vi "Agilent VNA Set Number of Points.vi"(6 "Channel":i8=1 min=1 max=99 step=1, 7 "Agilent VNA":T1, 8 "error in (no error)":errorcluster, 10 "Number Points":i32, 11 "VISA Resource Name":refnum<visa-resource-name>) -> (0 "error out":errorcluster, 3 "dup VISA Resource Name":refnum<visa-resource-name>)   [LabVIEW 2011]
doc: "This VI for the HP 8753B is used to read the number of stimulus points."
uses:
  TypeDefs/Agilent VNA Instrument Info.ctl
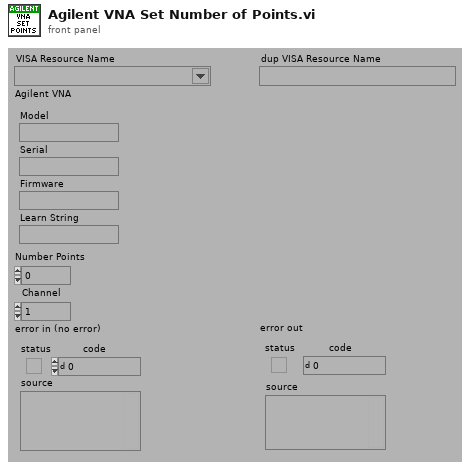
[diagram p1: front panel]
types:
  T1 = typedef "Agilent VNA Instrument Info.ctl" = cluster{"Model":string, "Serial":string, "Firmware":string, "Learn String":string}
  T2 = typedef "Agilent VNA Model.ctl" = enum16{"Not Supported", "8510X", "8719X", "8720X", "8722X", "8753X", "ENA", "PNA", "Field Fox"}
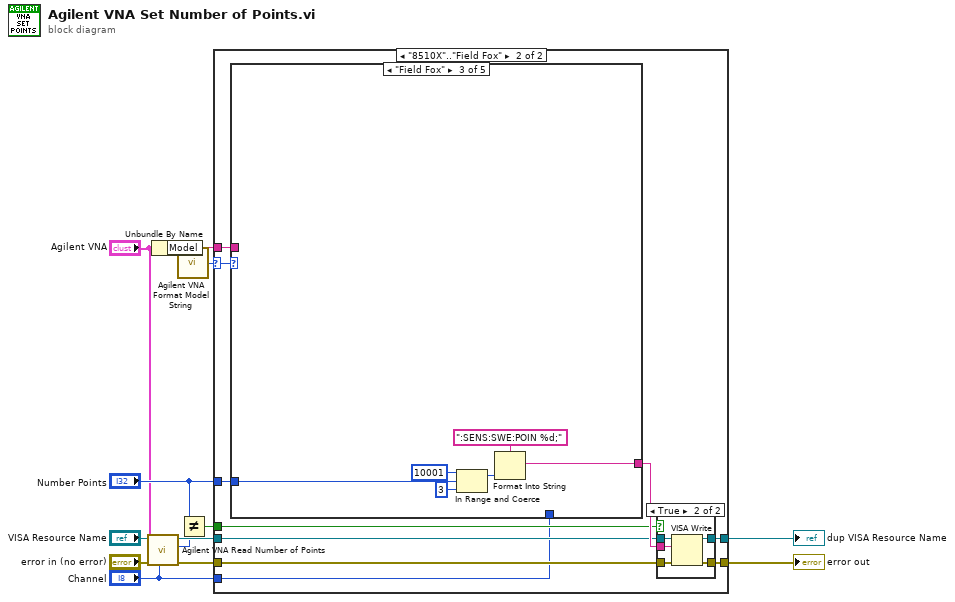
[diagram p0: block diagram]
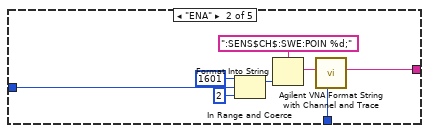
[diagram p4: hidden frame]
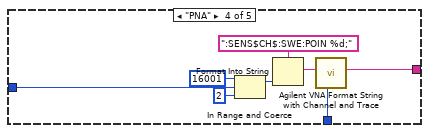
[diagram p5: hidden frame]
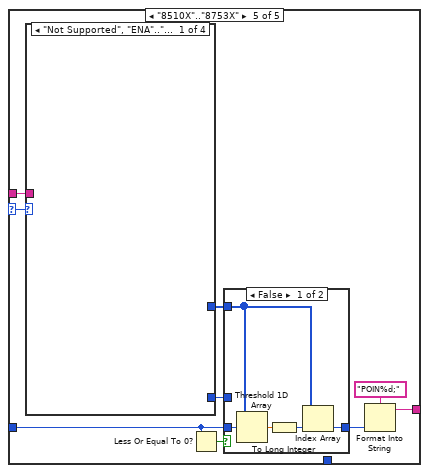
[diagram p6: hidden frame]
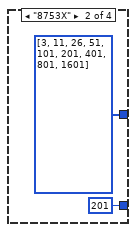
[diagram p8: hidden frame]
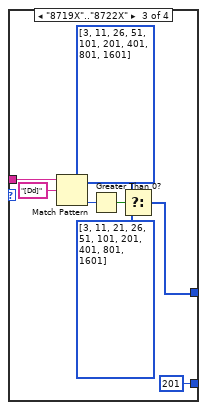
[diagram p9: hidden frame]
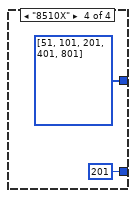
[diagram p10: hidden frame]
diagram:
  n1 = call "Agilent VNA Read Number of Points.vi"("Channel"="Channel", "Agilent VNA"="Agilent VNA", "error in (no error)"="error in (no error)", "VISA Resource Name"="VISA Resource Name") -> ("error out"=w6:errorcluster, "Number Points"=w5:i32, "dup VISA Resource Name"=w7:refnum<visa-resource-name>)  [unwired: 5 out]
  n2 = Unbundle By Name("Agilent VNA") -> ("Model"=w1:string)
  n3 = call "Agilent VNA Format Model String.vi"("Model"=w1) -> ("Model"=w2:T2)
  n4 = Not Equal?(x="Number Points", y=w5) -> (x != y?=w10:bool)
  n5 = case shown="\"8510X\"..\"Field Fox\"" w2 {
    selector: w2 -> [_ w17]
    tunnel: [w15 w25] -> w13
    tunnel: [w14 w24] -> w12
    tunnel: "Number Points" -> [_ w22]
    tunnel: w10 -> [_ w21]
    tunnel: w7 -> [w15 w20]
    tunnel: w6 -> [w14 w19]
    tunnel: "Channel" -> [_ w18]
    tunnel: w1 -> [_ w16]
    frame "Not Supported" {
    }
    frame "8510X".."Field Fox" {
      n6 = case shown="\"Field Fox\"" w17 {
        selector: w17 -> [_ _ _ _ w49]
        tunnel: [_ w27 w34 w41 w53] -> w23
        tunnel: w22 -> [_ w33 w39 w47 w50]
        tunnel: w18 -> [_ w26 _ w40 _]
        tunnel: w16 -> [_ _ _ _ w48]
        frame "Not Supported" {
        }
        frame "ENA" {
          n7 = In Range and Coerce(upper limit=1601, x=w33, lower limit=2) -> (coerced(x)=w29:i32)  [unwired: 1 out]
          n8 = Format Into String(format string=":SENS$CH$:SWE:POIN %d;", w29) -> (resulting string=w28:string)  [unwired: 2 in, 1 out]
          n9 = call "Agilent VNA Format String with Channel and Trace.vi"("Channel"=w26, "String"=w28) -> ("String Out"=w27:string)  [unwired: 1 in, 6 out]
        }
        frame "Field Fox" {
          n10 = In Range and Coerce(upper limit=10001, x=w39, lower limit=3) -> (coerced(x)=w35:i32)  [unwired: 1 out]
          n11 = Format Into String(format string=":SENS:SWE:POIN %d;", w35) -> (resulting string=w34:string)  [unwired: 2 in, 1 out]
        }
        frame "PNA" {
          n12 = In Range and Coerce(upper limit=16001, x=w47, lower limit=2) -> (coerced(x)=w43:i32)  [unwired: 1 out]
          n13 = Format Into String(format string=":SENS$CH$:SWE:POIN %d;", w43) -> (resulting string=w42:string)  [unwired: 2 in, 1 out]
          n14 = call "Agilent VNA Format String with Channel and Trace.vi"("Channel"=w40, "String"=w42) -> ("String Out"=w41:string)  [unwired: 1 in, 6 out]
        }
        frame "8510X".."8753X" {
          n15 = case shown="\"Not Supported\", \"ENA\"..\"Field Fox\"" w49 {
            tunnel: [_ i32[] [3, 11, 26, 51, 101, 201, 401, 801, 1601] w65 i32[] [51, 101, 201, 401, 801]] -> w55
            tunnel: [_ 201 201 201] -> w51
            tunnel: w48 -> [_ _ w70 _]
            frame "Not Supported", "ENA".."Field Fox" {
            }
            frame "8753X" {
            }
            frame "8719X".."8722X" {
              n16 = Match Pattern(string=w70, regular expression="[Dd]") -> (offset past match=w69:i32)  [unwired: 4 out]
              n17 = Greater Than 0?(x=w69) -> (x > 0?=w68:bool)
              n18 = Select(t=i32[] [3, 11, 26, 51, 101, 201, 401, 801, 1601], s=w68, f=i32[] [3, 11, 21, 26, 51, 101, 201, 401, 801, 1601]) -> (s? t:f=w65:i32[])
            }
            frame "8510X" {
            }
          }
          n19 = Less Or Equal To 0?(x=w50) -> (x <= 0?=w52:bool)
          n20 = case shown="False" w52 {
            tunnel: w55 -> [w60 _]
            tunnel: [w58 w62] -> w54
            tunnel: w50 -> [w57 _]
            tunnel: w51 -> [_ w62]
            frame False {
              n21 = Threshold 1D Array(2:w57, 3:w60) -> (0:w61:dbl)  [unwired: 1 out]
              n22 = To Long Integer(number=w61) -> (32bit integer=w59:i32)
              n23 = Index Array(array=w60, index=w59) -> (element=w58:i32)
            }
            frame True {
            }
          }
          n24 = Format Into String(format string="POIN%d;", w54) -> (resulting string=w53:string)  [unwired: 2 in, 1 out]
        }
      }
      n25 = case shown="True" w21 {
        tunnel: w20 -> [w76 w81]
        tunnel: w19 -> [w75 w80]
        tunnel: [w76 w79] -> w25
        tunnel: [w75 w78] -> w24
        tunnel: w23 -> [_ w77]
        frame False {
        }
        frame True {
          n26 = VISA Write(VISA resource name=w81, write buffer=w77, error in (no error)=w80) -> (VISA resource name out=w79:refnum<visa-resource-name>, error out=w78:errorcluster)  [unwired: 1 out]
        }
      }
    }
  }
  "dup VISA Resource Name" <- w13
  "error out" <- w12
